vi "USRP_freqsweepUSRP2.vi"() -> ()   [LabVIEW 2021]
uses:
  <vilib>/addons/Modulation/Analog/controls/Complex Data Waveform.ctl
  <vilib>/measure/maspectr.llb/Power Spectrum and PSD Export Mode.ctl
  system stop.vi
  <vilib>/measure/matone.llb/Extract Single Tone Information 1 Chan (CDB).vi
  <vilib>/measure/maspectr.llb/FFT Power Spectrum and PSD for 1 Chan (CDB).vi
  <instrlib>/niUSRP/niUSRP Fetch Rx Data (CDB Cluster).vi
  <instrlib>/niUSRP/niUSRP Write Tx Data (CDB Cluster).vi
  <vilib>/addons/Modulation/niAMT.lvlib
  <vilib>/measure/NI_MAPro.lvlib
panel:
  in  "Tab Control":T1(tab)
  in  "IQ rate":dbl=100000.0 format="%#_6p"
  in  "Tx Gain":dbl format="%#_6f"
  in  "Tx IP":refnum<k15>
  out "coerced IQ rate Tx":dbl=100000.0 format="%#_6p"
  out "coerced carrier frequency Tx":dbl=100000.0 format="%#_6p"
  in  "Rx IP":refnum<k15>
  in  "Rx gain":dbl format="%#_6f"
  in  "Frequency":dbl format="%#_13g"
  in  "Duration":dbl format="%#_13g"
  out "coerced IQ rate Rx":dbl=100000.0 format="%#_6p"
  out "coerced carrier frequency Rx":dbl=100000.0 format="%#_6p"
  in  "number of samples":i64=100000
  out "Waveform Graph":dbl[](graph)
  out "Received Waveform Graph":cluster{"f0":dbl, "df":dbl, "magnitude":dbl[]}(graph)
  out "detected frequency":dbl format="%.2p"
  out "detected Amplitude in dBm":dbl format="%.2p"
  out "Off":bool=TRUE
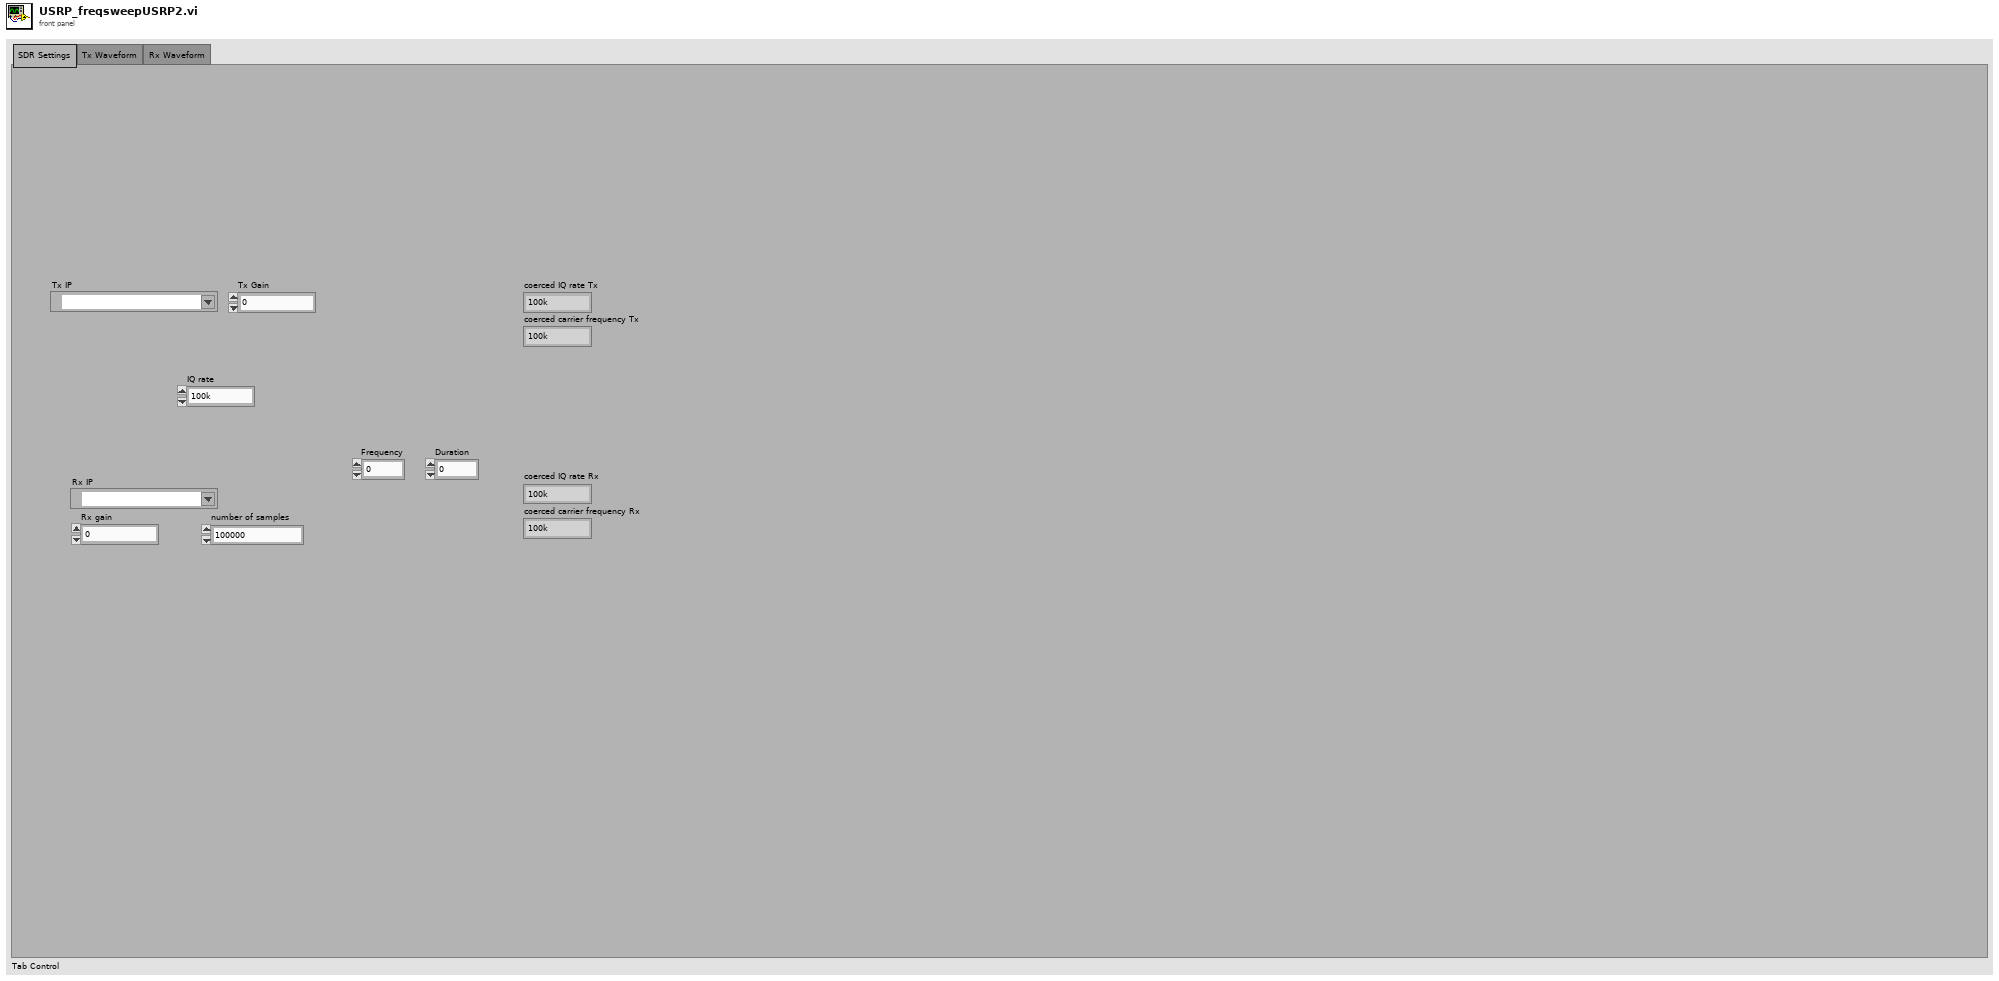
[diagram p1: front panel]
types:
  T1 = enum32{"SDR Settings", "Tx Waveform", "Rx Waveform"}
  T2 = typedef "niAMT.lvlib/Complex Data Waveform.ctl" = cluster{"t0":dbl, "dt":dbl, "Y":cdb[]}
  T3 = typedef "NI_MAPro.lvlib/Power Spectrum and PSD Export Mode.ctl" = u16
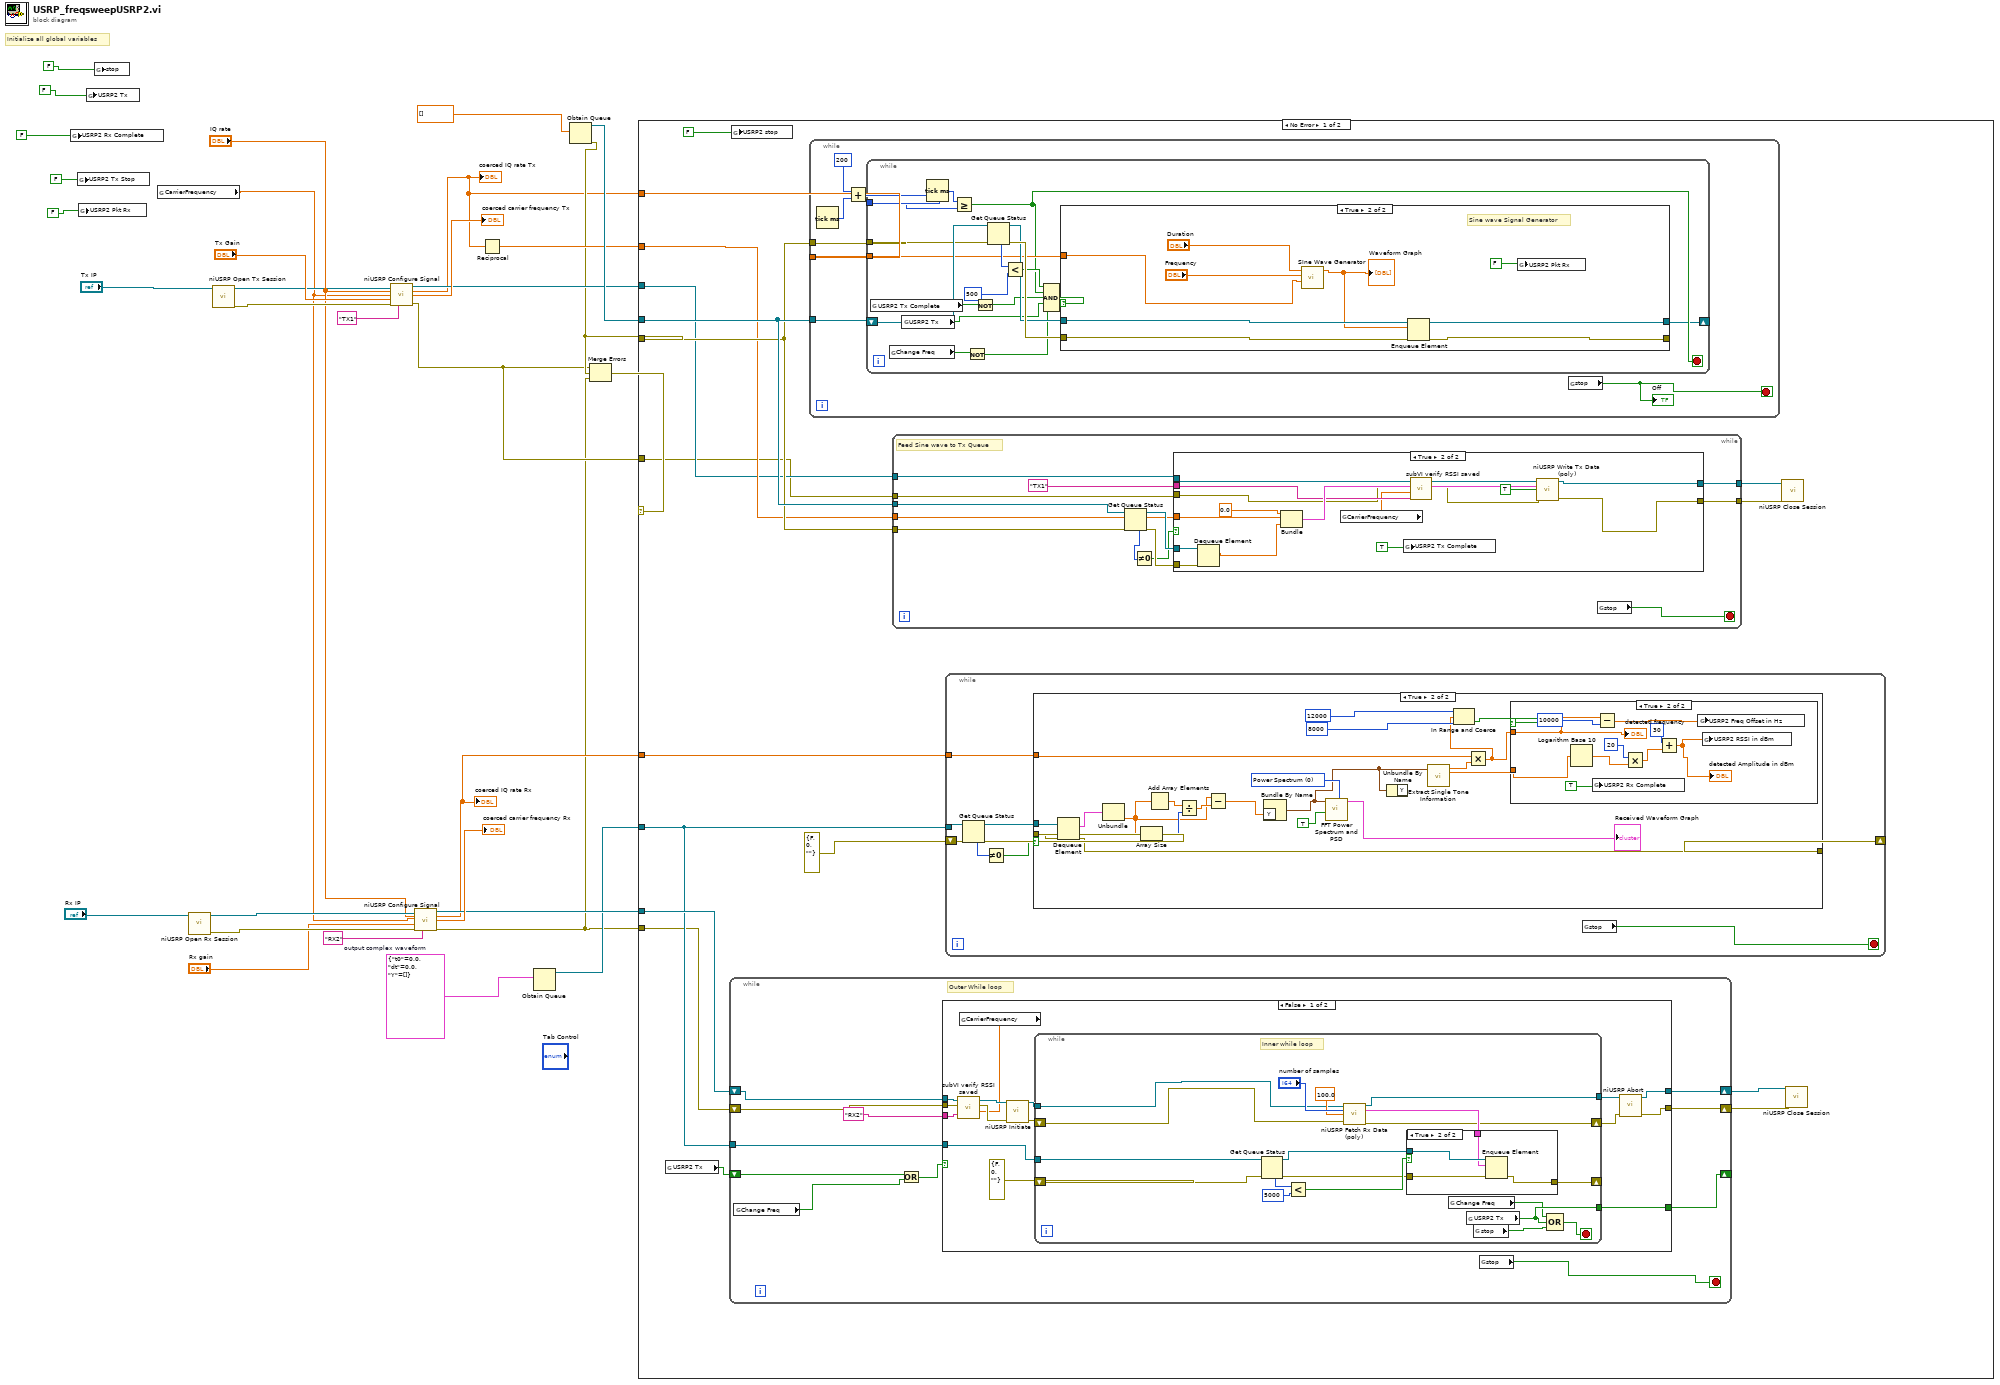
[diagram p0: block diagram]
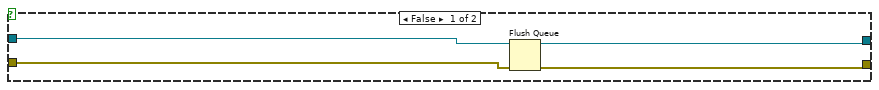
[diagram p2: hidden frame]
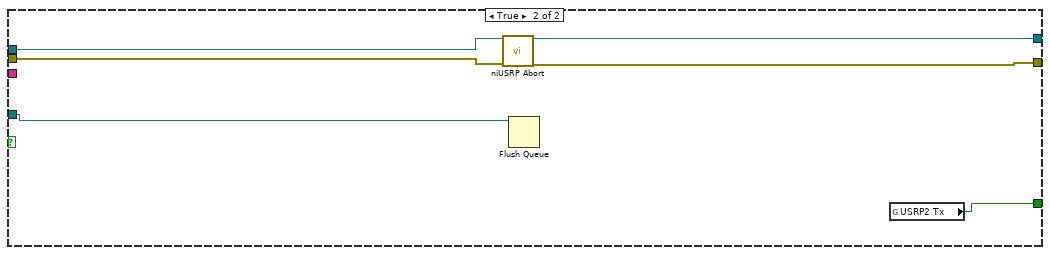
[diagram p4: hidden frame]
diagram:
  w6 = T2 {"t0"=0.0, "dt"=0.0, "Y"=[]}  # output complex waveform
  # "Initialize all global variables"
  n1 = global write "system stop.vi" "USRP2 Rx Complete"(FALSE) -> ()
  n2 = global write "system stop.vi" "USRP2 Tx Stop"(FALSE) -> ()
  n3 = global write "system stop.vi" "USRP2 Pkt Rx"(FALSE) -> ()
  n4 = global write "system stop.vi" "USRP2 Tx"(FALSE) -> ()
  n5 = global write "system stop.vi" "stop"(FALSE) -> ()
  n6 = global read "system stop.vi" "CarrierFrequency"() -> (w1:dbl)
  n7 = call <instrlib>:"niUSRP Open Rx Session.vi"("device names"="Rx IP") -> ("session handle out"=w26:refnum<k15>, "error out"=w25:errorcluster)  [unwired: 13 in]
  n8 = call <instrlib>:"niUSRP Open Tx Session.vi"("device names"="Tx IP") -> ("session handle out"=w30:refnum<k15>, "error out"=w29:errorcluster)  [unwired: 13 in]
  n9 = call <instrlib>:"niUSRP Configure Signal.vi"("session handle"=w30, "IQ rate"="IQ rate", "carrier frequency"=w1, "gain"="Tx Gain", "error in (no error)"=w29, "active antenna"="TX1") -> ("session handle out"=w13:refnum<k15>, "coerced IQ rate"=w10:dbl, "coerced carrier frequency"=→"coerced carrier frequency Tx":dbl, "error out"=w9:errorcluster)  [unwired: 5 in, 1 out]
  "coerced IQ rate Tx" <- w10
  n10 = call <instrlib>:"niUSRP Configure Signal.vi"("session handle"=w26, "IQ rate"="IQ rate", "carrier frequency"=w1, "gain"="Rx gain", "error in (no error)"=w25, "active antenna"="RX2") -> ("session handle out"=w7:refnum<k15>, "coerced IQ rate"=w4:dbl, "coerced carrier frequency"=→"coerced carrier frequency Rx":dbl, "error out"=w2:errorcluster)  [unwired: 5 in, 1 out]
  "coerced IQ rate Rx" <- w4
  n11 = Reciprocal(x=w10) -> (1/x=w12:dbl)
  n12 = Obtain Queue(element data type=w6) -> (queue out=w5:refnum<queue>)  [unwired: 4 in, 2 out]
  n13 = Obtain Queue(element data type=dbl[] []) -> (queue out=w14:refnum<queue>, error out=w11:errorcluster)  [unwired: 4 in, 1 out]
  n14 = Merge Errors(w9, w11, w2) -> (w16:errorcluster)
  n15 = case shown="No Error" w16 {
    tunnel: w11 -> [w48 _]
    tunnel: w14 -> [w49 _]
    tunnel: w13 -> [w46 _]
    tunnel: w12 -> [w47 _]
    tunnel: w10 -> [w45 _]
    tunnel: w9 -> [w44 _]
    tunnel: w7 -> [w42 _]
    tunnel: w5 -> [w41 _]
    tunnel: w4 -> [w40 _]
    tunnel: w2 -> [w39 _]
    frame No Error {
      n16 = global read "system stop.vi" "USRP2 Tx"() -> (w33:bool)
      n17 = while {
        tunnel: w41 -> [w98]
        shift-right: [w97] -> w37
        shift-left: w42 -> [w88]
        shift-right: [w96] -> w36
        shift-left: w39 -> [w89]
        shift-right: [w92] -> _
        shift-left: w33 -> [w93]
        stop <- w95 stop-if-true
        # "Outer While loop"
        n18 = global read "system stop.vi" "Change Freq"() -> (w91:bool)
        n19 = Or(x=w93, y=w91) -> (x .or. y?=w94:bool)
        n20 = case shown="False" w94 {
          tunnel: w98 -> [w113 w141]
          tunnel: [w108 w143] -> w97
          tunnel: [w107 w142] -> w96
          tunnel: [w105 w140] -> w92
          tunnel: "RX2" ("Configuration:Active Antenna") -> [w104 _]
          tunnel: w89 -> [w103 w138]
          tunnel: w88 -> [w102 w139]
          frame False {
            n21 = global read "system stop.vi" "CarrierFrequency"() -> (w99:dbl)
            n22 = call "subVI verify RSSI saved.vi"("Configuration:Active Antenna"=w104, "Configuration:Carrier Frequency"=w99, "error in (no error)"=w103, "reference"=w102) -> ("error out"=w101:errorcluster, "reference out"=w100:refnum<k15>)  [unwired: 6 in]
            n23 = call <instrlib>:"niUSRP Initiate.vi"("session handle"=w100, "error in (no error)"=w101) -> ("session handle out"=w111:refnum<k15>, "error out"=w110:errorcluster)  [unwired: 12 in]
            n24 = while {
              tunnel: w113 -> [w132]
              shift-right: [w119] -> w106
              shift-left: w110 -> [w117]
              shift-right: [w131] -> _
              shift-left: errorcluster {"status"=FALSE, "code"=0, "source"=""} ("error in (no error)") -> [w130]
              tunnel: w111 -> [w118]
              tunnel: [w120] -> w109
              tunnel: [w115] -> w105
              stop <- w122 stop-if-true
              # "Inner while loop"
              n25 = Get Queue Status(queue=w132, error in (no error)=w130) -> (queue out=w125:refnum<queue>, error out=w126:errorcluster, # elements in queue=w129:i32)  [unwired: 1 in, 5 out]
              n26 = Less?(x=w129, y=5000) -> (x < y?=w127:bool)
              n27 = call-poly <instrlib>:"niUSRP Fetch Rx Data (poly).vi"("session handle"=w118, "number of samples"="number of samples", "timeout"=100.0, "error in (no error)"=w117) -> ("session handle out"=w120:refnum<k15>, "data"=w123:cluster{"t0":dbl, "dt":dbl, "Y":cdb[]}, "error out"=w119:errorcluster)  [unwired: 8 in, 1 out]
              n28 = case shown="True" w127 {
                tunnel: w126 -> [w133 w137]
                tunnel: w125 -> [_ w136]
                tunnel: w123 -> [_ w135]
                tunnel: [w133 w134] -> w131
                frame False {
                }
                frame True {
                  n29 = Enqueue Element(queue=w136, element=w135, error in (no error)=w137) -> (error out=w134:errorcluster)  [unwired: 1 in, 2 out]
                }
              }
              n30 = global read "system stop.vi" "Change Freq"() -> (w114:bool)
              n31 = global read "system stop.vi" "USRP2 Tx"() -> (w115:bool)
              n32 = global read "system stop.vi" "stop"() -> (w116:bool)
              n33 = Compound Arithmetic op=OR(w114, w115, w116) -> (w122:bool)
            }
            n34 = call <instrlib>:"niUSRP Abort.vi"("session handle"=w109, "error in (no error)"=w106) -> ("session handle out"=w108:refnum<k15>, "error out"=w107:errorcluster)  [unwired: 12 in]
          }
          frame True {
            n35 = call <instrlib>:"niUSRP Abort.vi"("session handle"=w139, "error in (no error)"=w138) -> ("session handle out"=w143:refnum<k15>, "error out"=w142:errorcluster)  [unwired: 12 in]
            n36 = Flush Queue(queue=w141) -> ()  [unwired: 1 in, 3 out]
            n37 = global read "system stop.vi" "USRP2 Tx"() -> (w140:bool)
          }
        }
        n38 = global read "system stop.vi" "stop"() -> (w95:bool)
      }
      n39 = global write "system stop.vi" "USRP2 stop"(FALSE) -> ()
      n40 = while {
        tunnel: w49 -> [w56]
        tunnel: w48 -> [w55]
        tunnel: w45 -> [w54]
        stop <- w50 stop-if-true
        n41 = Tick Count (ms)() -> (millisecond timer value=w53:u32)
        n42 = Add(x=200, y=w53) -> (x+y=w52:u32)
        n43 = while {
          tunnel: w55 -> [w69]
          tunnel: w54 -> [w68]
          tunnel: w52 -> [w63]
          shift-right: [w59] -> _
          shift-left: w56 -> [w70]
          stop <- w62 stop-if-true
          n44 = global read "system stop.vi" "USRP2 Tx Complete"() -> (w61:bool)
          n45 = global read "system stop.vi" "Change Freq"() -> (w58:bool)
          n46 = global read "system stop.vi" "USRP2 Tx"() -> (w66:bool)
          n47 = Tick Count (ms)() -> (millisecond timer value=w64:u32)
          n48 = Greater Or Equal?(x=w64, y=w63) -> (x >= y?=w62:bool)
          n49 = Not(x=w58) -> (.not. x?=w57:bool)
          n50 = Not(x=w61) -> (.not. x?=w60:bool)
          n51 = Get Queue Status(queue=w70, error in (no error)=w69) -> (queue out=w71:refnum<queue>, error out=w72:errorcluster, # elements in queue=w74:i32)  [unwired: 1 in, 5 out]
          n52 = Less?(x=w74, y=500) -> (x < y?=w67:bool)
          n53 = Compound Arithmetic op=AND(w67, w62, w60, w66, w57) -> (w65:bool)
          n54 = case shown="True" w65 {
            tunnel: w72 -> [w77 w87]
            tunnel: w71 -> [w78 w86]
            tunnel: [w76 w85] -> w59
            tunnel: [w75 w84] -> _
            tunnel: w68 -> [_ w81]
            frame False {
              n55 = Flush Queue(queue=w78, error in (no error)=w77) -> (queue out=w76:refnum<queue>, error out=w75:errorcluster)  [unwired: 1 out]
            }
            frame True {
              # "Sine wave Signal Generator"
              n56 = call "SIne Wave Generator.vi"("Sampling rate"=w81, "Frequency"="Frequency", "Duration"="Duration") -> ("Array"=w80:dbl[])  [unwired: 7 in, 1 out]
              "Waveform Graph" <- w80
              n57 = Enqueue Element(queue=w86, element=w80, error in (no error)=w87) -> (queue out=w85:refnum<queue>, error out=w84:errorcluster)  [unwired: 1 in, 1 out]
              n58 = global write "system stop.vi" "USRP2 Pkt Rx"(FALSE) -> ()
            }
          }
        }
        n59 = global read "system stop.vi" "stop"() -> (w50:bool)
        "Off" <- w50
      }
      n60 = while {
        tunnel: w49 -> [w196]
        tunnel: w48 -> [w193]
        tunnel: w47 -> [w192]
        tunnel: w46 -> [w185]
        tunnel: w44 -> [w184]
        tunnel: [w189] -> w35
        tunnel: [w188] -> w34
        stop <- w187 stop-if-true
        # "Feed Sine wave to Tx Queue"
        n61 = Get Queue Status(queue=w196, error in (no error)=w193) -> (queue out=w195:refnum<queue>, error out=w194:errorcluster, # elements in queue=w191:i32)  [unwired: 1 in, 5 out]
        n62 = Not Equal To 0?(x=w191) -> (x != 0?=w190:bool)
        n63 = case shown="True" w190 {
          tunnel: w195 -> [_ w214]
          tunnel: w194 -> [_ w213]
          tunnel: w192 -> [_ w212]
          tunnel: w185 -> [w198 w199]
          tunnel: w184 -> [w197 w202]
          tunnel: [w198 w207] -> w189
          tunnel: [w197 w205] -> w188
          tunnel: "TX1" ("Configuration:Active Antenna") -> [_ w204]
          frame False {
          }
          frame True {
            n64 = Dequeue Element(queue=w214, error in (no error)=w213) -> (element=w210:dbl[])  [unwired: 1 in, 3 out]
            n65 = Bundle(0.0, w212, w210) -> (w211:cluster{dbl, dbl, dbl[]})  [unwired: 1 in]
            n66 = global read "system stop.vi" "CarrierFrequency"() -> (w200:dbl)
            n67 = global write "system stop.vi" "USRP2 Tx Complete"(TRUE) -> ()
            n68 = call "subVI verify RSSI saved.vi"("Configuration:Active Antenna"=w204, "Configuration:Carrier Frequency"=w200, "error in (no error)"=w202, "reference"=w199) -> ("error out"=w203:errorcluster, "reference out"=w201:refnum<k15>)  [unwired: 6 in]
            n69 = call-poly <instrlib>:"niUSRP Write Tx Data (poly).vi"("session handle"=w201, "data"=w211, "end of data?"=TRUE, "error in (no error)"=w203) -> ("session handle out"=w207:refnum<k15>, "error out"=w205:errorcluster)  [unwired: 10 in]
          }
        }
        n70 = global read "system stop.vi" "stop"() -> (w187:bool)
      }
      n71 = while {
        tunnel: w41 -> [w149]
        shift-right: [w146] -> _
        shift-left: errorcluster {"status"=FALSE, "code"=0, "source"=""} ("error in (no error)") -> [w148]
        tunnel: w40 -> [w145]
        stop <- w144 stop-if-true
        n72 = Get Queue Status(queue=w149, error in (no error)=w148) -> (queue out=w151:refnum<queue>, error out=w150:errorcluster, # elements in queue=w152:i32)  [unwired: 1 in, 5 out]
        n73 = Not Equal To 0?(x=w152) -> (x != 0?=w147:bool)
        n74 = case shown="True" w147 {
          tunnel: w151 -> [_ w173]
          tunnel: w150 -> [w153 w167]
          tunnel: [w153 w165] -> w146
          tunnel: w145 -> [_ w164]
          frame False {
          }
          frame True {
            w170 = T3 0 items=["Power Spectrum", "Power Spectral Density"] ("export mode")
            n75 = Dequeue Element(queue=w173, error in (no error)=w167) -> (element=w166:T2, error out=w165:errorcluster)  [unwired: 1 in, 2 out]
            n76 = Unbundle(w166) -> ("Y"=w160:cdb[])  [unwired: 2 out]
            n77 = Array Size(array=w160) -> (size(s)=w162:i32)
            n78 = Add Array Elements(numeric array=w160) -> (sum=w163:cdb)
            n79 = Divide(x=w163, y=w162) -> (x/y=w161:cdb)
            n80 = Subtract(x=w160, y=w161) -> (x-y=w159:cdb[])
            n81 = Bundle By Name("Y"=w159) -> (w168:waveform(cdb))  [unwired: 1 in]
            n82 = call-poly <vilib>:"FFT Power Spectrum and PSD.vi"("export mode"=w170, "dB On (F)"=TRUE, "time signal"=w168) -> ("Power Spectrum / PSD"=→"Received Waveform Graph":cluster{"f0":dbl, "df":dbl, "magnitude":dbl[]})  [unwired: 5 in, 3 out]
            n83 = Unbundle By Name(w168) -> ()  [unwired: 1 out]
            n84 = call-poly <vilib>:"Extract Single Tone Information.vi"("time signal in"=w168) -> ("detected amplitude"=w154:dbl, "detected frequency"=w169:dbl)  [unwired: 5 in, 4 out]
            n85 = Multiply(x=w164, y=w169) -> (x*y=w155:dbl)
            n86 = In Range and Coerce(upper limit=12000, x=w155, lower limit=8000) -> (In Range?=w156:bool)  [unwired: 1 out]
            n87 = case shown="True" w156 {
              tunnel: w155 -> [_ w176]
              tunnel: w154 -> [_ w183]
              frame False {
              }
              frame True {
                n88 = Logarithm Base 10(1:w183) -> (0:w181:dbl)
                n89 = global write "system stop.vi" "USRP2 Rx Complete"(TRUE) -> ()
                n90 = Subtract(x=w176, y=10000) -> (x-y=w174:dbl)
                n91 = Multiply(x=20, y=w181) -> (x*y=w179:dbl)
                n92 = Add(x=30, y=w179) -> (x+y=w177:dbl)
                "detected Amplitude in dBm" <- w177
                n93 = global write "system stop.vi" "USRP2 Freq Offset in Hz"(w174) -> ()
                n94 = global write "system stop.vi" "USRP2 RSSI in dBm"(w177) -> ()
                "detected frequency" <- w176
              }
            }
          }
        }
        n95 = global read "system stop.vi" "stop"() -> (w144:bool)
      }
      n96 = call <instrlib>:"niUSRP Close Session.vi"("session handle"=w35, "error in (no error)"=w34) -> ()  [unwired: 13 in, 1 out]
      n97 = call <instrlib>:"niUSRP Close Session.vi"("session handle"=w37, "error in (no error)"=w36) -> ()  [unwired: 13 in, 1 out]
    }
    frame Error {
    }
  }
